vi "isRecording.vi"(0 "Camera in":refnum<class "Camera.lvclass">, 11 "error in (no error)":errorcluster) -> (4 "Camera out":refnum<class "Camera.lvclass">, 6 "recording":bool, 15 "error out":errorcluster)   [LabVIEW 2020, in "Camera.lvclass"]
doc: "Retreive the rec handle.\nThis handle allows direct access to all underlying functions of the pco.recorder."
uses:
  Camera.lvclass
  Camera.lvclass/Camera.ctl
  Recorder.lvlib
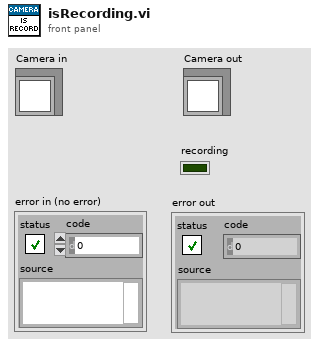
[diagram p1: front panel]
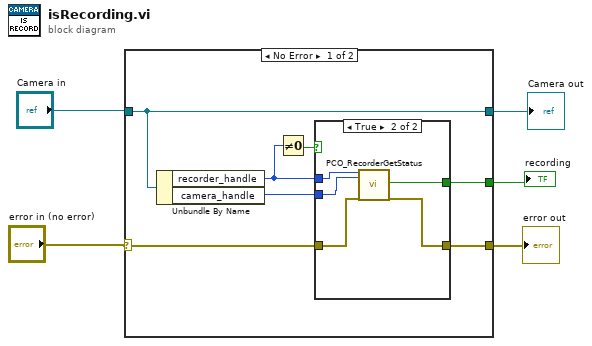
[diagram p0: block diagram]
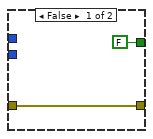
[diagram p2: hidden frame]
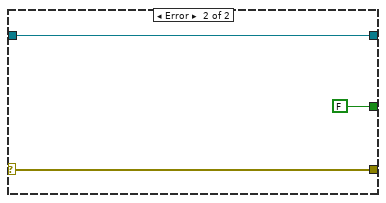
[diagram p3: hidden frame]
diagram:
  n1 = case shown="No Error" "error in (no error)" {
    selector: "error in (no error)" -> [w9 w22]
    tunnel: [w8 w22] -> w3
    tunnel: [w12 w21] -> w4
    tunnel: "Camera in" -> [w12 w21]
    tunnel: [w10 FALSE] -> w1
    frame No Error {
      n2 = Unbundle By Name(w12) -> ("recorder_handle"=w7:u64, "camera_handle"=w11:u64)
      n3 = Not Equal To 0?(x=w7) -> (x != 0?=w6:bool)
      n4 = case shown="True" w6 {
        tunnel: w11 -> [_ w19]
        tunnel: [FALSE ("bIsRunning") w18] -> w10
        tunnel: w9 -> [w13 w17]
        tunnel: [w13 w16] -> w8
        tunnel: w7 -> [_ w15]
        frame False {
        }
        frame True {
          n5 = call "PCO_RecorderGetStatus.vi"("phRec"=w15, "phCam"=w19, "error in (no error)"=w17) -> ("bIsRunning"=w18:bool, "error out"=w16:errorcluster)  [unwired: 5 in, 10 out]
        }
      }
    }
    frame Error {
    }
  }
  "error out" <- w3
  "Camera out" <- w4
  "recording" <- w1
